vi "Set Controller .NET.vi"(10 "ControllerBase":refnum<k24>, 11 "ControllerBase in":refnum<class "ControllerBase.lvclass">) -> (3 "ControllerBase out":refnum<class "ControllerBase.lvclass">)   [LabVIEW 2025, in "ControllerBase.lvclass"]
uses:
  ControllerBase.lvclass
  D:/git/Sourcegrid-LabVIEW/dll/SourceGrid.dll
  dll/SourceGrid.dll
  ControllerBase.lvclass/ControllerBase.ctl
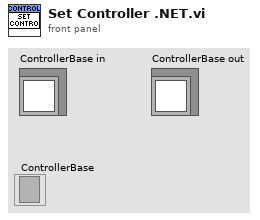
[diagram p1: front panel]
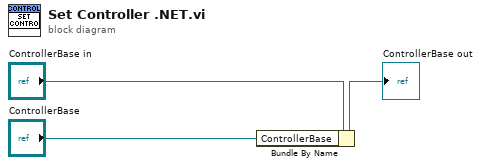
[diagram p0: block diagram]
diagram:
  n1 = Bundle By Name(cluster="ControllerBase in", "ControllerBase"="ControllerBase") -> (→"ControllerBase out":refnum<class "ControllerBase.lvclass">)
